vi "AmpPolNames_DG535.vi"(0 "Polarity array":refnum<vi>[](array[refnum]), 1 "Amplitude array":refnum<vi>[](array[refnum])) -> (2 "Array 2":enum16{"Negative", "Positive"}[](array[ring]), 3 "Array 3":dbl[](array[numeric]), 4 "Array 4":string[](array[string]), 5 "Array":string[][](array[string]))   [LabVIEW 2013]
uses:
  Device Drivers/DG645/subVIs/polarity_TypDEf.ctl
panel:
  out "Array 6":string[](array[string])
  out "Array 5":T1[](array[typedef])
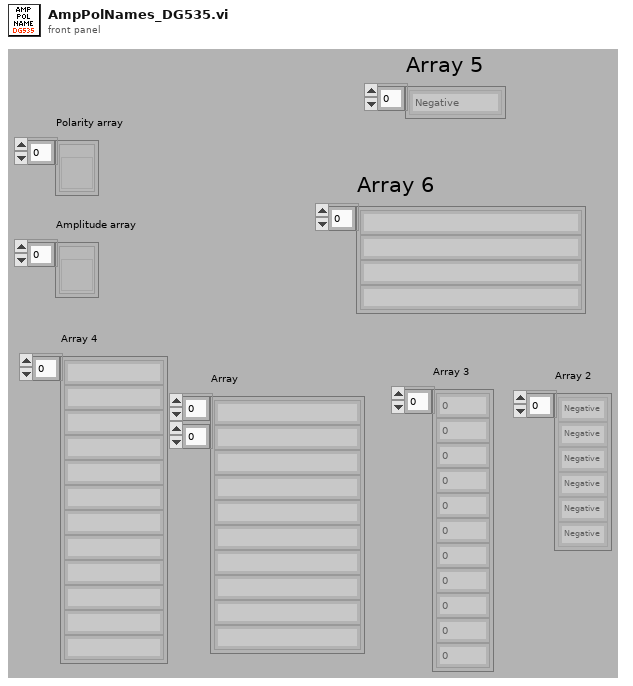
[diagram p1: front panel]
types:
  T1 = typedef "polarity_TypDEf.ctl" = enum16{"Negative", "Positive"}
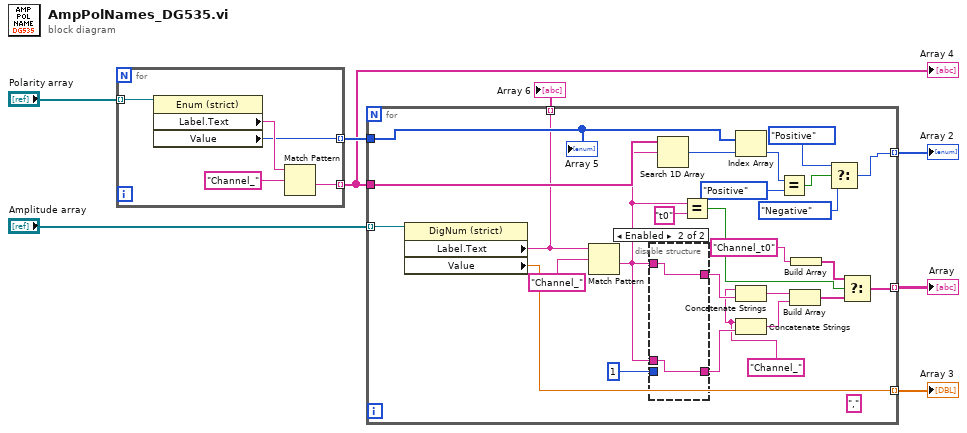
[diagram p0: block diagram]
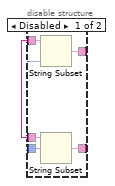
[diagram p2: hidden frame]
diagram:
  n1 = for {
    tunnel: "Polarity array" -> [w13] mode=indexing
    tunnel: [w10] -> w3 mode=indexing
    tunnel: [w9] -> w4 mode=indexing
    n2 = property class="Enum (strict)"(reference=w13) -> ("Label.Text"=w11:string, "Value"=w9:enum16{"Negative", "Positive"})  [unwired: 1 in, 2 out]
    n3 = Match Pattern(string=w11, regular expression="Channel_") -> (after substring=w10:string)  [unwired: 1 in, 3 out]
  }
  "Array 4" <- w3
  n4 = for {
    tunnel: "Amplitude array" -> [w39] mode=indexing
    tunnel: [w33] -> w7 mode=indexing
    tunnel: [w26] -> w5 mode=indexing
    tunnel: w3 -> [w25]
    tunnel: w4 -> [w24]
    tunnel: [w17] -> w6 mode=indexing
    tunnel: [w16] -> w1 mode=indexing
    w15 = "Channel_" ("string")
    (unwired) "," ("string")
    n5 = property class="DigNum (strict)"(reference=w39) -> ("Label.Text"=w16:string, "Value"=w26:dbl)  [unwired: 1 in, 2 out]
    n6 = Match Pattern(string=w16, regular expression="Channel_") -> (after substring=w14:string)  [unwired: 1 in, 3 out]
    n7 = disable-structure shown="Enabled" {
      disable-tunnel: 1 ("offset (0)") -> [w43 _]
      disable-tunnel: [w42 w45] -> w34
      disable-tunnel: [w41 w44] -> w30
      disable-tunnel: w14 -> [w40 w44]
      disable-tunnel: w14 -> [_ w45]
      frame Disabled {
        n8 = String Subset(string=w40, length (rest)=w43) -> (substring=w42:string)  [unwired: 1 in]
        n9 = String Subset(string=w40, offset (0)=w43) -> (substring=w41:string)  [unwired: 1 in]
      }
      frame Enabled {
      }
    }
    n10 = Search 1D Array(1D array=w25, element=w14) -> (index of element=w23:i32)  [unwired: 1 in]
    n11 = Equal?(x=w14, y="t0") -> (x = y?=w37:bool)
    n12 = Index Array(array=w24, index=w23) -> (element=w22:enum16{"Negative", "Positive"})
    n13 = Concatenate Strings(w15, w34) -> (w28:string)
    n14 = Concatenate Strings(w15, w30) -> (w27:string)
    n15 = Equal?(x=w22, y=polarity_TypDEf."Positive") -> (x = y?=w20:bool)
    n16 = Build Array(w28, w27) -> (w29:string[])
    n17 = Build Array("Channel_t0" ("t")) -> (w31:string[])
    n18 = Select(t=polarity_TypDEf."Positive" ("y"), s=w20, f=polarity_TypDEf."Negative" ("y")) -> (s? t:f=w17:T1)
    n19 = Select(t=w31, s=w37, f=w29) -> (s? t:f=w33:string[])
    "Array 5" <- w24
  }
  "Array" <- w7
  "Array 2" <- w6
  "Array 3" <- w5
  "Array 6" <- w1
